vi "Test 1 Move Into Pipe.vi"(8 "error in (no error)":errorcluster, 11 "Test Case In":refnum<class "Day X Test.lvclass">) -> (0 "error out":errorcluster, 3 "Test Case Out":refnum<class "Day X Test.lvclass">)   [LabVIEW 2020, in "Day X Test.lvclass"]
uses:
  Day X Test.lvclass
  Day X Test.lvclass/Day X Test.ctl
  4993e8ee-a06a-463a-9684-69129f64d5ce.vi
  Map/Map.lvclass
  Map/Position.ctl
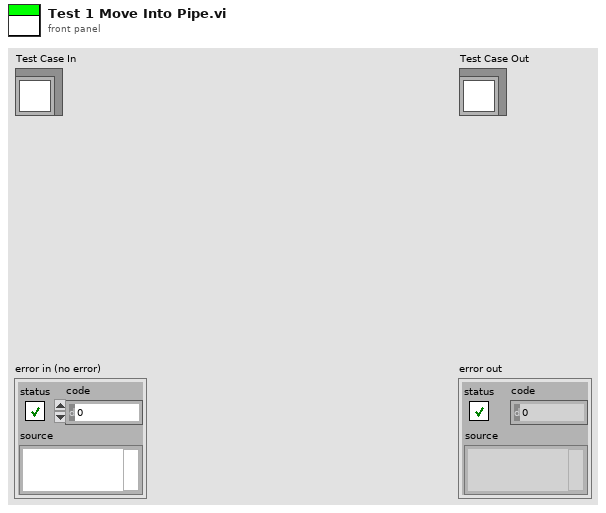
[diagram p1: front panel]
types:
  T1 = typedef "Map.lvclass/Position.ctl" = cluster{"Row":u64, "Col":u64, "Next Move":enum16{"North", "East", "South", "West", "Halt"}}
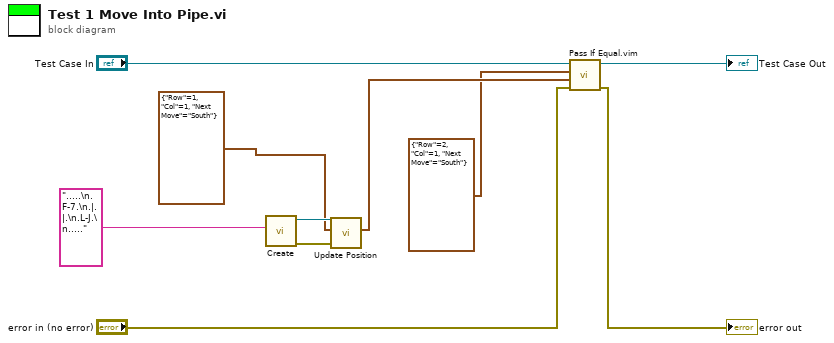
[diagram p0: block diagram]
diagram:
  n1 = call "Create.vi"("Input"=".....\n.F-7.\n.|.|.\n.L-J.\n.....") -> ("error out"=w4:errorcluster, "Map"=w5:refnum<class "Map.lvclass">)  [unwired: 9 in]
  n2 = call "Update Position.vi"("error in (no error)"=w4, "Current"=T1 {"Row"=1, "Col"=1, "Next Move"=enum."South"}, "Map In"=w5) -> ("Next"=w2:T1)  [unwired: 6 in, 2 out]
  n3 = call "Pass If Equal.vim"("error in (no error)"="error in (no error)", "Actual"=w2, "Expected"=T1 {"Row"=2, "Col"=1, "Next Move"=enum."South"}, "LUnit Test Case In"="Test Case In") -> ("error out"=→"error out":errorcluster, "LUnit Test Case Out"=→"Test Case Out":refnum<class "Day X Test.lvclass">)  [unwired: 6 in]
